vi "construct_configure_rf.vi"(0 "port":enum16{"rx", "tx"}(ring), 5 "fc (Hz)":dbl format="%#_6p", 7 "gain (dB)":dbl, 11 "error in (no error)":errorcluster) -> (4 "command out":T2=enum."configure_rf", 6 "parameters JSON":string, 10 "data out":variant, 14 "Debug info":string, 15 "error out":errorcluster)   [LabVIEW 2019, in "mmW_commands.lvlib"]
uses:
  mmW_commands.lvlib
  TypeDefs/commands.ctl
  TypeDefs/_depr_datatypes.ctl
  configure_rf.ctl
  <vilib>/addons/_JKI.lib/Serialization/JSON/JKI JSON Serialization.lvlib
panel:
  out "datatype (only for debug)":T1
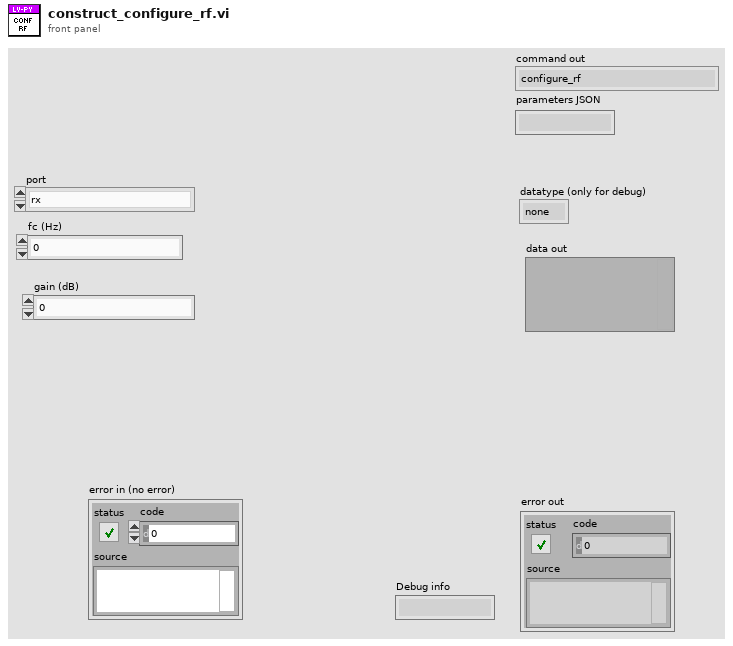
[diagram p1: front panel]
types:
  T1 = typedef "mmW_commands.lvlib/_depr_datatypes.ctl" = enum16{"none", "float", "string", "CSG_wfm", "DBL_wfm"}
  T2 = typedef "mmW_commands.lvlib/commands.ctl" = enum16{"configure_fs", "configure_rf", "configure_trigger", "equalization_enable", "equalization_start", "lo_sync_enable", "equalization_stop", "get_instrument_status", "get_versions", "initialize_hw", "pop_rx", "set_log_level", "Shutdown", "start", "start_instrument_app", "stop", "trans", "transceive", "trigger_burst", "trigger_sync_enable", "Write TX", "resp_generic", "resp_waveform", "send_trigger", "fetch", "transceive2"}
  T3 = typedef "mmW_commands.lvlib/configure_rf.ctl" = cluster{"port":enum16{"rx", "tx"}, "fc":dbl, "gain":dbl, "datatype":string}
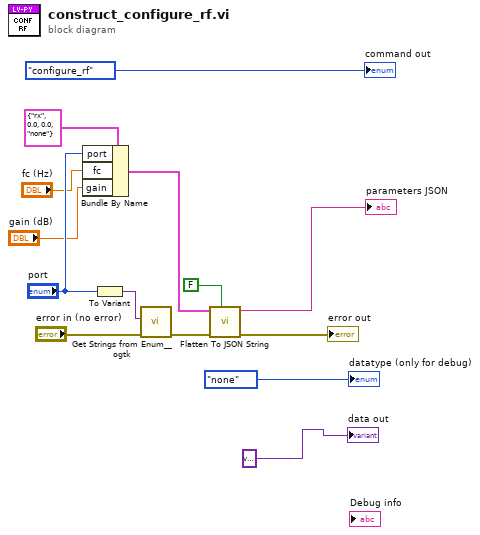
[diagram p0: block diagram]
diagram:
  n1 = Bundle By Name(cluster=T3 {"port"=enum."rx", "fc"=0.0, "gain"=0.0, "datatype"="none"} ("Cluster"), "port"="port", "fc"="fc (Hz)", "gain"="gain (dB)") -> (w6:T3)
  n2 = To Variant(anything="port") -> (Variant=w14:variant)
  n3 = call <userlib>:"Get Strings from Enum__ogtk.vi"("error in (no error)"="error in (no error)", "Enum"=w14) -> ("error out"=w9:errorcluster)  [unwired: 6 in, 3 out]
  n4 = call <vilib>:"Flatten To JSON String.vi"("Multiline (T)"=FALSE, "error in (no error)"=w9, "Variant"=w6) -> ("error out"=→"error out":errorcluster, "JSON String"=→"parameters JSON":string)  [unwired: 7 in]
  "command out" <- commands."configure_rf" ("mmW_instrument_commands")
  "datatype (only for debug)" <- _depr_datatypes."none" ("datatypes")
  "data out" <- variant
